vi "main.vi"() -> ()   [LabVIEW 2020, in "main.lvlib"]
uses:
  main.lvlib
  vars.ctl
  <vilib>/DAQmx/read.llb/DAQmx Read (Analog 1D Wfm NChan NSamp).vi
  <vilib>/NI/AMC/Read Termination Message.vi
  <vilib>/NI/AMC/Create Single Message.vi
  <vilib>/NI/AMC/Update Message Routing Info.vi
  _queueName.vi
  <vilib>/NI/AMC/Globals.vi
  <vilib>/NI/AMC/Send Message.vi
  <vilib>/DAQmx/configure/timing.llb/DAQmx Timing (Sample Clock).vi
  <vilib>/DAQmx/miscellaneous.llb/DAQmx Fill In Error Info.vi
  <vilib>/NI/AMC/AMC.lvlib
panel:
  out "Ceravac":dbl(knob) scale=0.0..150.0
  in  "sampling":u8=1 caption="sampling interval" min=1 max=10 format="%.0f s"
  out "saving?":bool
  in  "save":bool
  out "chart":dbl[][](graph)=[[111539.40736451437]]
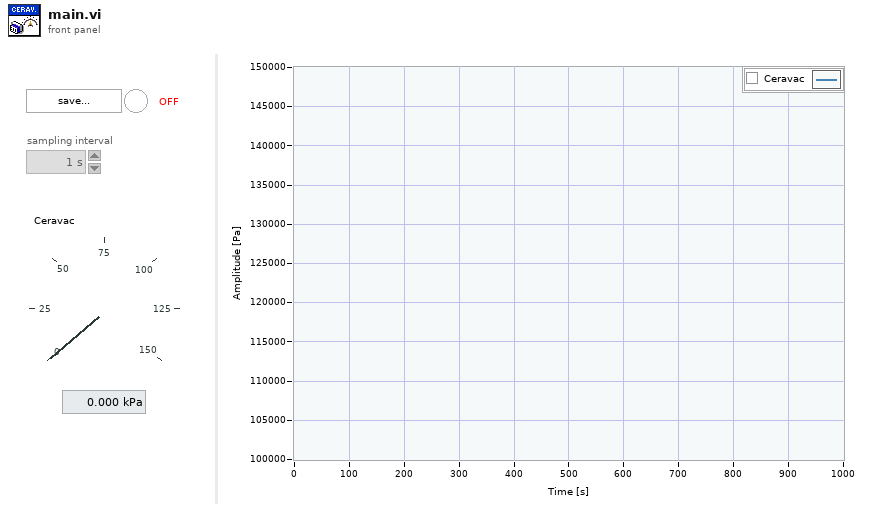
[diagram p1: front panel]
types:
  T1 = typedef "main.lvlib/vars.ctl" = cluster{"rate":dbl, "channel":refnum<k21>, "sample mode":i32, "task":refnum<k21>, "data":dynamicdata}
  T2 = typedef "AMC.lvlib/Message Queue.ctl" = refnum<queue>
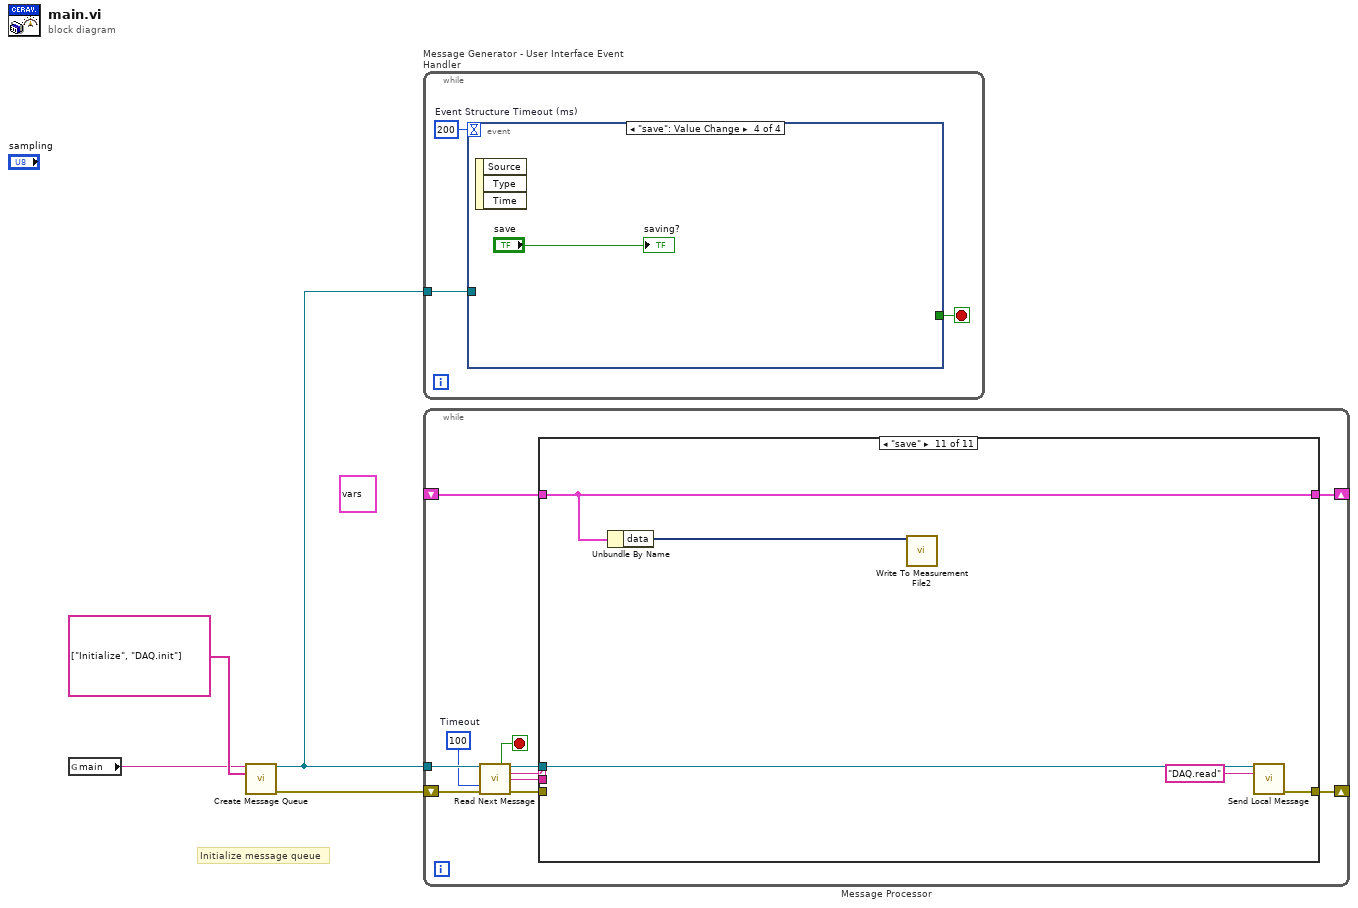
[diagram p0: block diagram]
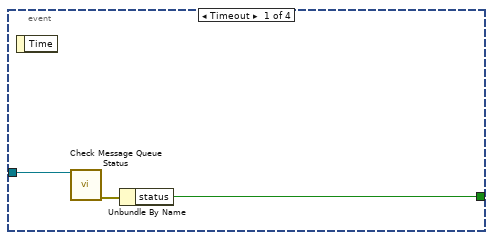
[diagram p2: hidden frame]
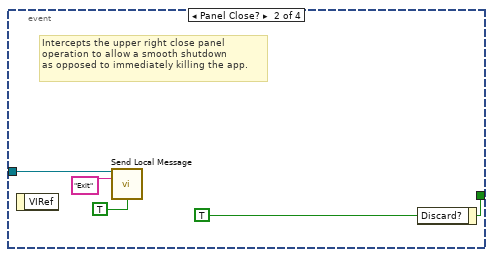
[diagram p3: hidden frame]
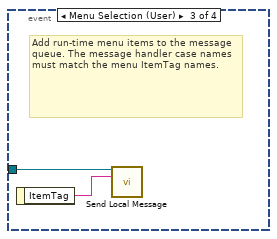
[diagram p4: hidden frame]
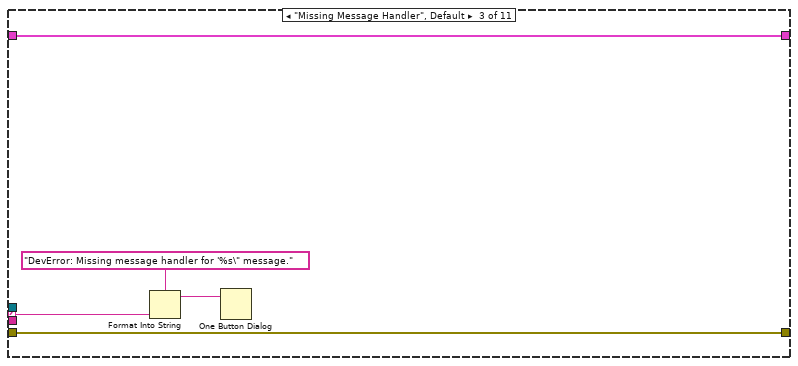
[diagram p7: hidden frame]
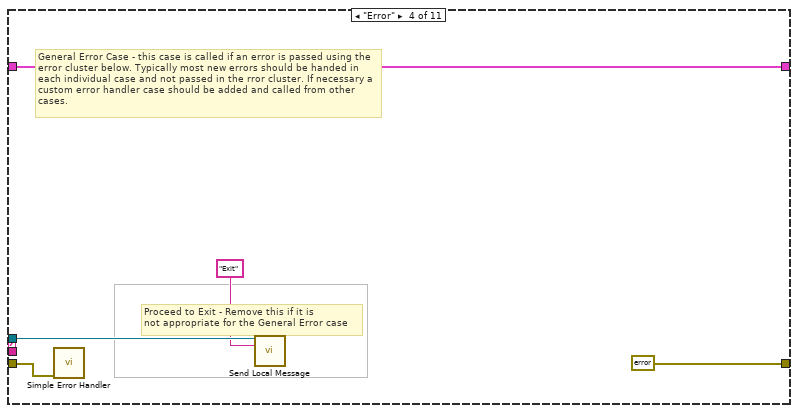
[diagram p8: hidden frame]
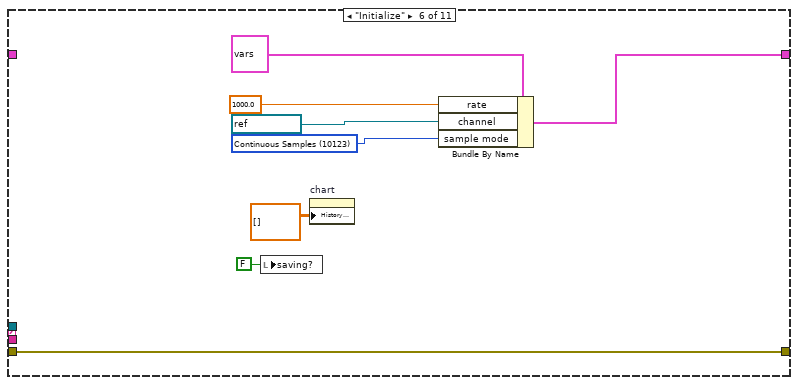
[diagram p10: hidden frame]
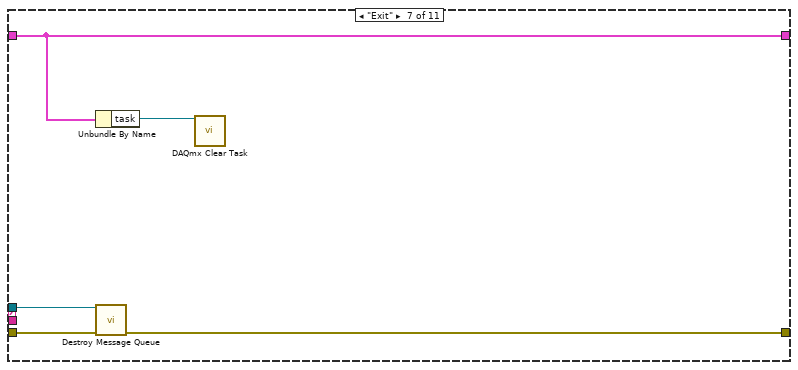
[diagram p11: hidden frame]
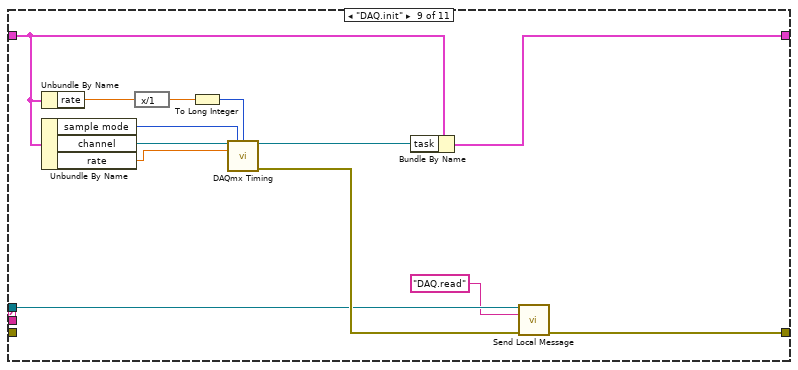
[diagram p13: hidden frame]
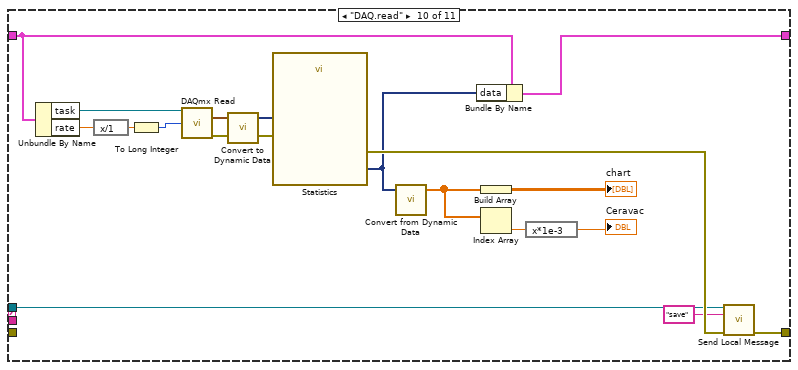
[diagram p14: hidden frame]
diagram:
  (unwired) T1 {"rate"=1000.0, "channel"="Ceravac", "sample mode"=10123, "task"="", "data"=[]} ("state variables")
  # "Initialize message queue"
  n1 = global read "_queueName.vi" "main"() -> (w1:string)
  n2 = call <vilib>:"Create Message Queue.vi"("message queue name"=w1, "initial message names"=string[] ["Initialize", "DAQ.init"]) -> ("message queue out"=w3:T2, "error out"=w2:errorcluster)  [unwired: 12 in]
  n3 = while "Message Generator - User Interface Event Handler" {
    tunnel: w3 -> [w5]
    stop <- w6 stop-if-true
    w7 = 200  # Event Structure Timeout (ms)
    n4 = event shown="[3] \"save\": Value Change" {
      selector: _ -> [_ _ _ _]
      dyn-events: _ -> [_ _ _ _]
      timeout: w7 -> [_ _ _ _]
      tunnel: [w8 w14 _ _] -> w6
      tunnel: w5 -> [w9 w12 w15 _]
      event Timeout {
        n5 = event-data() -> ()  [unwired: 2 out]
        n6 = call <vilib>:"Check Message Queue Status.vi"("message queue in"=w9) -> ("error out"=w10:errorcluster)  [unwired: 10 in, 4 out]
        n7 = Unbundle By Name(w10) -> ("status"=w8:bool)
      }
      event Panel Close? {
        w14 = TRUE ("Discard?")
        # "Intercepts the upper right close panel\noperation to allow a smooth shutdown\nas opposed to immediately killing the app."
        n8 = event-data() -> ()  [unwired: 2 out]
        n9 = call <vilib>:"Send Local Message.vi"("message queue in"=w12, "message name"="Exit", "priority message (F)"=TRUE) -> ()  [unwired: 10 in, 3 out]
        n10 = event-data("Discard?"=w14) -> ()  [unwired: 1 in, 1 out]
      }
      event Menu Selection (User) {
        # "Add run-time menu items to the message\nqueue. The message handler case names must match the menu ItemTag names."
        n11 = event-data() -> ("ItemTag"=w16:string)  [unwired: 1 out]
        n12 = call <vilib>:"Send Local Message.vi"("message queue in"=w15, "message name"=w16) -> ()  [unwired: 11 in, 3 out]
      }
      event "save": Value Change {
        n13 = event-data() -> ()  [unwired: 4 out]
        "saving?" <- "save"
      }
    }
  }
  n14 = while "Message Processor" {
    shift-left: w2 -> [w22]
    shift-right: [w26] -> _
    tunnel: w3 -> [w23]
    shift-left: _ -> [w28]
    shift-right: [w27] -> _
    stop <- w25 stop-if-true
    w18 = 100  # Timeout
    n15 = call <vilib>:"Read Next Message.vi"("message queue in"=w23, "timeout (1 ms)"=w18, "error in"=w22) -> ("exit process?"=w25:bool, "message queue out"=w24:T2, "message name"=w20:string, "message value"=w19:string, "error out"=w21:errorcluster)  [unwired: 5 in, 3 out]
    n16 = case shown="\"save\"" w20 {
      selector: w20 -> [_ _ w35 _ _ _ _ _ _ _ _]
      tunnel: [w30 w32 w37 w42 w44 w47 w54 w59 w65 w74 w92] -> w27
      tunnel: w28 -> [w30 w32 w37 w42 w44 _ w54 w59 w64 w73 w92]
      tunnel: w24 -> [_ _ _ w40 _ _ w56 _ w61 w83 w94]
      tunnel: w21 -> [w29 w31 w36 w38 w43 w52 w57 w58 _ _ _]
      tunnel: [w29 w31 w36 errorcluster {"status"=FALSE, "code"=0, "source"=""} ("error out") w43 w52 w55 w58 w62 w84 w95] -> w26
      tunnel: w19 -> [_ _ _ _ _ _ _ _ _ _ _]
      frame "---------- Framework Operations ----------" {
        # "Dummy case to add a seperator in the Case Structure menu"
      }
      frame "", "Idle" {
      }
      frame "Missing Message Handler", Default {
        n17 = Format Into String(format string="DevError: Missing message handler for '%s\" message." ("message"), w35) -> (resulting string=w33:string)  [unwired: 2 in, 1 out]
        n18 = One Button Dialog(message=w33) -> ()  [unwired: 2 out]
      }
      frame "Error" {
        # "Proceed to Exit - Remove this if it is\nnot appropriate for the General Error case"
        # "General Error Case - this case is called if an error is passed using the error cluster below. Typically most new errors should be handed in each individual case and not passed in the rror cluster. If necessary a custom error handler case should be added and called from other cases."
        n19 = call <vilib>:"Simple Error Handler.vi"("error in (no error)"=w38) -> ()  [unwired: 1 in, 8 out]
        n20 = call <vilib>:"Send Local Message.vi"("message queue in"=w40, "message name"="Exit") -> ()  [unwired: 11 in, 3 out]
      }
      frame "---------- Generic Operations ----------" {
        # "Dummy case to add a seperator in the Case Structure menu"
      }
      frame "Initialize" {
        w49 = 10123 items=["Finite Samples"=10178, "Continuous Samples"=10123, "Hardware Timed Single Point"=12522] ("sample mode")
        n21 = local write "saving?"(FALSE ("saving?")) -> ()
        n22 = property on="chart" class="WFChart (strict)"("History Data"=dbl[][] []) -> ()  [unwired: 2 in, 2 out]
        n23 = Bundle By Name(cluster=T1 {"rate"=1000.0, "channel"="Ceravac", "sample mode"=10123, "task"="", "data"=[]} ("state variables"), "rate"=1000.0, "channel"=refnum<k21> "Ceravac" ("DAQmx Global Channel"), "sample mode"=w49) -> (w47:T1)
      }
      frame "Exit" {
        n24 = Unbundle By Name(w54) -> ("task"=w53:refnum<k21>)
        n25 = call <vilib>:"Destroy Message Queue.vi"("message queue in"=w56, "error in"=w57) -> ("error out"=w55:errorcluster)  [unwired: 11 in, 2 out]
        n26 = call <vilib>:"DAQmx Clear Task.vi"("task in"=w53) -> ()  [unwired: 14 in, 1 out]
      }
      frame "---------- Application Operations ----------" {
      }
      frame "DAQ.init" {
        n27 = Unbundle By Name(w64) -> ("rate"=w69:dbl)
        n28 = Unbundle By Name(w64) -> ("sample mode"=w70:i32, "channel"=w72:refnum<k21>, "rate"=w71:dbl)
        n29 = expression code="x/1"(w69) -> (w68:dbl)
        n30 = To Long Integer(number=w68) -> (32bit integer=w67:i32)
        n31 = call-poly <vilib>:"DAQmx Timing.vi"("task/channels in"=w72, "sample mode"=w70, "samples per channel"=w67, "rate"=w71) -> ("task out"=w66:refnum<k21>, "error out"=w63:errorcluster)  [unwired: 10 in]
        n32 = Bundle By Name(cluster=w64, "task"=w66) -> (w65:T1)
        n33 = call <vilib>:"Send Local Message.vi"("message queue in"=w61, "message name"="DAQ.read", "error in"=w63) -> ("error out"=w62:errorcluster)  [unwired: 10 in, 2 out]
      }
      frame "DAQ.read" {
        n34 = Unbundle By Name(w73) -> ("task"=w90:refnum<k21>, "rate"=w79:dbl)
        n35 = expression code="x/1"(w79) -> (w81:dbl)
        n36 = To Long Integer(number=w81) -> (32bit integer=w80:i32)
        n37 = call-poly <vilib>:"DAQmx Read.vi"("task/channels in"=w90, "number of samples per channel"=w80) -> ("data"=w87:waveform(dbl)[], "error out"=w89:errorcluster)  [unwired: 11 in, 1 out]
        n38 = call "Convert to Dynamic Data"("Array of Waveforms"=w87) -> ("Dynamic Data Type"=w86:dynamicdata)  [unwired: 3 in]
        n39 = call "Statistics"("Signals"=w86, "error in (no error)"=w89) -> ("Arithmetic Mean"=w75:dynamicdata, "error out"=w88:errorcluster)  [unwired: 24 in]
        n40 = call "Convert from Dynamic Data"("Dynamic Data Type"=w75) -> ("Array"=w77:dbl[])  [unwired: 3 in]
        n41 = Bundle By Name(cluster=w73, "data"=w75) -> (w74:T1)
        n42 = Build Array(w77) -> (→"chart":dbl[][])
        n43 = Index Array(array=w77) -> (element=w78:dbl)  [unwired: 1 in]
        n44 = expression code="x*1e-3"(w78) -> (→"Ceravac":dbl)
        n45 = call <vilib>:"Send Local Message.vi"("message queue in"=w83, "message name"="save", "error in"=w88) -> ("error out"=w84:errorcluster)  [unwired: 10 in, 2 out]
      }
      frame "save" {
        n46 = Unbundle By Name(w92) -> ("data"=w91:dynamicdata)
        n47 = call "Write To Measurement File2"("Signals"=w91) -> ()  [unwired: 16 in, 3 out]
        n48 = call <vilib>:"Send Local Message.vi"("message queue in"=w94, "message name"="DAQ.read") -> ("error out"=w95:errorcluster)  [unwired: 11 in, 2 out]
      }
    }
  }
